vi "Send Analogues.vi"() -> ()   [LabVIEW 2023]
uses:
  <vilib>/rvi/interface/nirviReadWriteControl/nirviReadWriteControl.xnode
  NiFpgaLv.dll
  <vilib>/Utility/error.llb/Error Cluster From Error Code.vi
  <vilib>/rvi/interface/Simulation/niFpgaSimulationCallBeginRW.vi
  <vilib>/rvi/errors/niLvFpgaAdjustHostInterfaceError.vi
  <vilib>/rvi/interface/nirviMethod/nirviMethod.xnode
  <vilib>/FPGAPlugInAG/Dynamic/niLvFpga_WriteFifo_Dynamic.vi
  <vilib>/rvi/errors/niLvFpgaMergeErrorWithErrorCode.vi
panel:
  in  "FPGA VI Reference In":refnum<k20>
  in  "TCP error in":errorcluster
  out "connection ID out":refnum<k5>
  in  "connection ID in":refnum<k5>
  out "data out 200":string
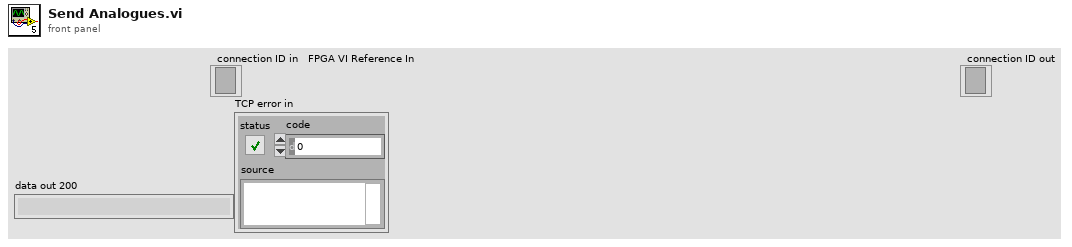
[diagram p1: front panel]
types:
  T1 = enum16{"Standard", "Buffered", "CRLF", "Immediate"}
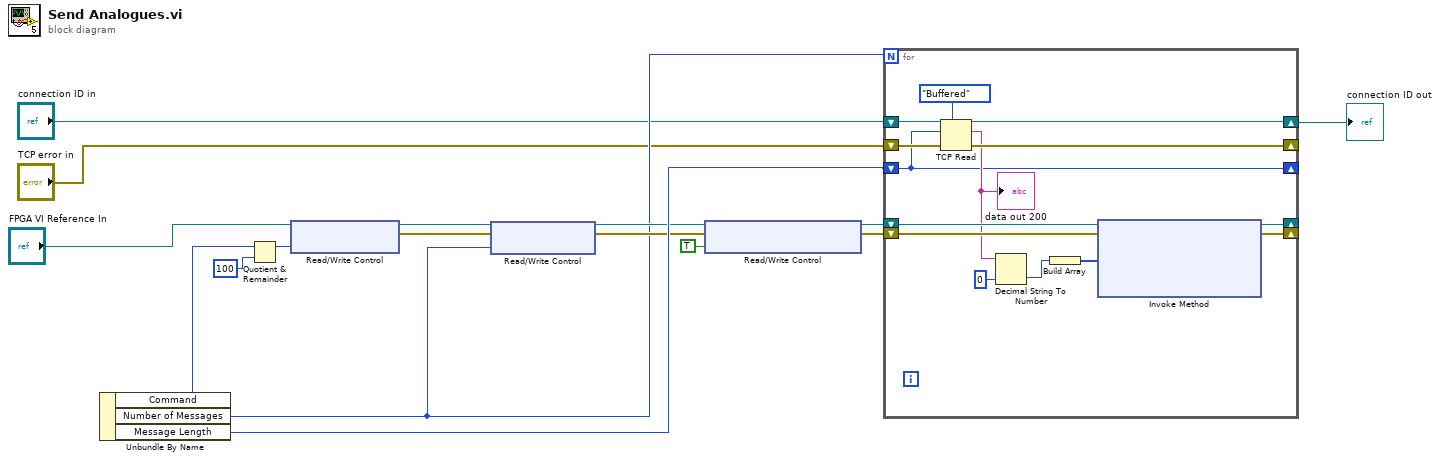
[diagram p0: block diagram]
diagram:
  n1 = Unbundle By Name() -> ("Command"=w14:u16, "Number of Messages"=w5:u32, "Message Length"=w17:u16)  [unwired: 1 in]
  n2 = Quotient & Remainder(x=w14, y=u8 100) -> (x-y*floor(x/y)=w12:u16)  [unwired: 1 out]
  n3 = xnode "Read/Write Control"("FPGA VI Reference In"="FPGA VI Reference In", "Memory to Write"=w12) -> ("FPGA VI Reference Out"=w7:refnum<k20>, "error in"=w10:errorcluster, "error out"=w9:errorcluster)
  n4 = xnode "Read/Write Control"("FPGA VI Reference In"=w7, "error in"=w9, "Nr of Analogues"=w5) -> ("FPGA VI Reference Out"=w6:refnum<k20>, "error out"=w8:errorcluster)
  n5 = xnode "Read/Write Control"("FPGA VI Reference In"=w6, "error in"=w8, "Trigger analogues transfer"=TRUE) -> ("FPGA VI Reference Out"=w16:refnum<k20>, "error out"=w15:errorcluster)
  n6 = for {
    N: w5 -> [_]
    shift-right: [w31] -> _
    shift-left: "TCP error in" -> [w26]
    shift-right: [w30] -> w3
    shift-left: "connection ID in" -> [w27]
    shift-right: [w18] -> _
    shift-left: w17 -> [w18]
    shift-right: [w29] -> _
    shift-left: w16 -> [w23]
    shift-right: [w24] -> _
    shift-left: w15 -> [w28]
    n7 = TCP Read(connection ID=w27, bytes to read=w18, error in (no error)=w26, 7:T1."Buffered" ("mode (standard)")) -> (connection ID out=w30:refnum<k5>, data out=w22:string, error out=w31:errorcluster)  [unwired: 1 in]
    "data out 200" <- w22
    n8 = Decimal String To Number(string=w22, default (0L)=u64 0 ("default (0 I32)")) -> (number=w19:u64)  [unwired: 1 in, 1 out]
    n9 = Build Array(w19) -> (w20:u64[])
    n10 = xnode "Invoke Method"("FPGA VI Reference In"=w23, "error in"=w28, "Data"=w20) -> ("FPGA VI Reference Out"=w29:refnum<k20>, "error out"=w24:errorcluster)  [unwired: 1 in, 1 out]
  }
  "connection ID out" <- w3
